vi "frontp_launch_default_subpanels.vi"(8 "error in (no error)":errorcluster, 11 "front_panel in":refnum<class "front_panel.lvclass">) -> (0 "error out":errorcluster, 3 "front_panel out":refnum<class "front_panel.lvclass">)   [LabVIEW 2015, in "front_panel.lvclass"]
uses:
  front_panel.lvclass
  Hardware Class/hardware_panel/Hardware_panel.lvclass
  hardware_caller_queue_numbers.ctl
  Detector_Class/detector_panel/Detector_panel.lvclass
  front_panel.lvclass/front_panel.ctl
  panel_class/panel.lvclass/panel.ctl
  panel_class/panel.lvclass
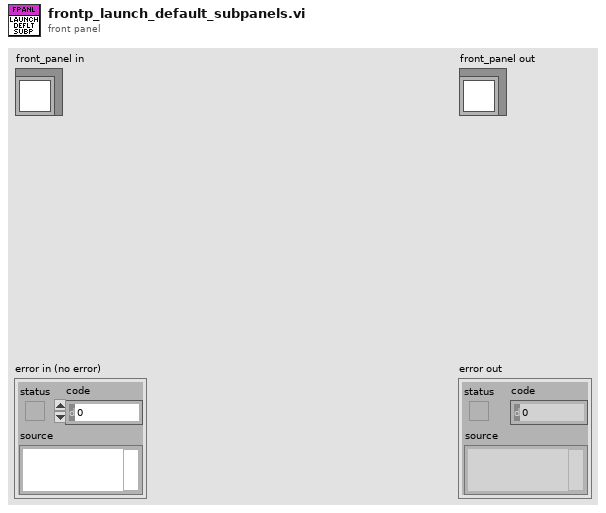
[diagram p1: front panel]
types:
  T1 = typedef "hardware_caller_queue_numbers.ctl" = enum16{"stage1", "stage2", "experiment", "detector"}
  T2 = typedef "gui_subpanel_references.ctl" = cluster{"Stage 1":refnum<vi>, "Stage 2":refnum<vi>, "Experiment":refnum<vi>, "Detector":refnum<vi>}
  T3 = typedef "hardware_seqs.ctl" = refnum<queue>[]
  T4 = typedef "ui_plot_references.ctl" = cluster{"plots":refnum<vi>, "chart":refnum<vi>, "graph":refnum<vi>, "map":refnum<vi>, "XY Graph":refnum<vi>}
  T5 = typedef "ui_user_events.ctl" = cluster{"update_xy_graph":refnum<user-event>, "update_graph":refnum<user-event>, "update_chart":refnum<user-event>, "update_map":refnum<user-event>, "event_loop_stop":refnum<user-event>, "keep_map":refnum<user-event>}
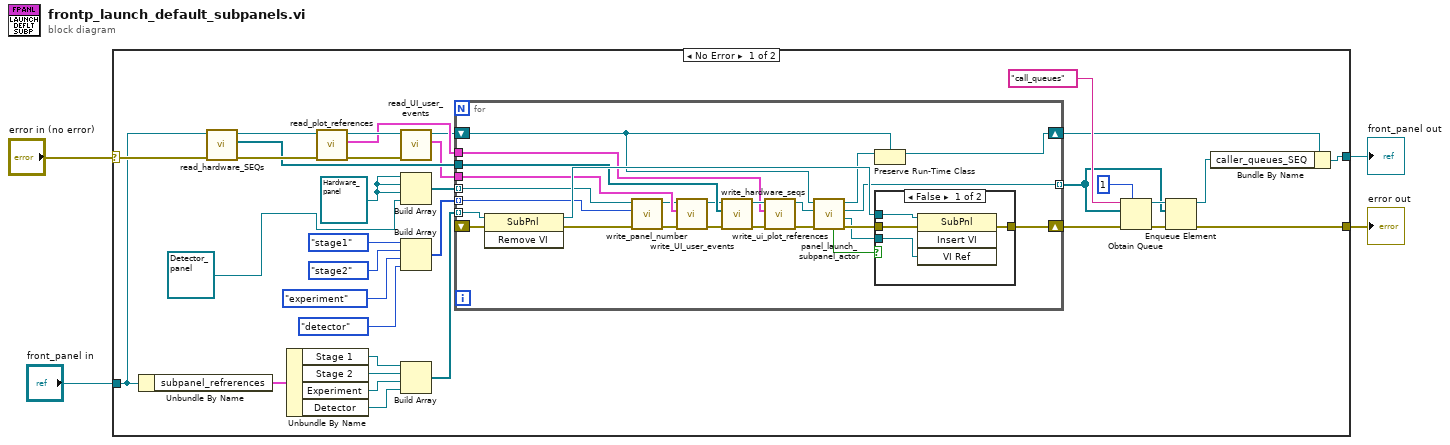
[diagram p0: block diagram]
diagram:
  n1 = case shown="No Error" "error in (no error)" {
    selector: "error in (no error)" -> [w15 w70]
    tunnel: [w26 w70] -> w3
    tunnel: [w28 w69] -> w1
    tunnel: "front_panel in" -> [w14 w69]
    frame No Error {
      w16 = refnum<class "Hardware_panel.lvclass"> refnum ("Hardware.lvclass")
      n2 = Unbundle By Name(w14) -> ("subpanel_refrerences"=w38:T2)
      n3 = call "read_hardware_SEQs.vi"("error in (no error)"=w15, "panel in"=w14) -> ("error out"=w13:errorcluster, "hardware_SEQs"=w9:T3, "panel out"=w12:refnum<class "front_panel.lvclass">)  [unwired: 7 in]
      n4 = Unbundle By Name(w38) -> ("Stage 1"=w37:refnum<vi>, "Stage 2"=w36:refnum<vi>, "Experiment"=w35:refnum<vi>, "Detector"=w34:refnum<vi>)
      n5 = call "read_plot_references.vi"("error in (no error)"=w13, "panel in"=w12) -> ("error out"=w10:errorcluster, "plot_references"=w8:T4, "panel out"=w11:refnum<class "front_panel.lvclass">)  [unwired: 7 in]
      n6 = call "read_UI_user_events.vi"("error in (no error)"=w10, "panel in"=w11) -> ("ui_user_events"=w7:T5, "panel out"=w6:refnum<class "front_panel.lvclass">)  [unwired: 7 in, 1 out]
      n7 = Build Array(w16, w16, w16, refnum<class "Detector_panel.lvclass"> refnum ("Detector_panel.lvclass")) -> (w17:refnum<class "panel.lvclass">[])
      n8 = Build Array(hardware_caller_queue_numbers."stage1" ("panel_number"), hardware_caller_queue_numbers."stage2" ("element"), hardware_caller_queue_numbers."experiment" ("element"), hardware_caller_queue_numbers."detector" ("element")) -> (w18:T1[])
      n9 = Build Array(w37, w36, w35, w34) -> (w33:refnum<vi>[])
      n10 = for {
        tunnel: w33 -> [w63] mode=indexing
        shift-right: [w60] -> w30
        shift-left: _ -> [w62]
        tunnel: w17 -> [w41] mode=indexing
        shift-right: [w53] -> w29
        shift-left: w6 -> [w54]
        tunnel: [w58] -> w24 mode=indexing
        tunnel: w9 -> [w47]
        tunnel: w18 -> [w39] mode=indexing
        tunnel: w8 -> [w48]
        tunnel: w7 -> [w44]
        n11 = invoke class="SubPnl" method="Remove VI"(reference=w63, error in=w62) -> (reference out=w61:refnum<vi>, error out=w43:errorcluster)  [unwired: 1 in, 1 out]
        n12 = call "write_panel_number.vi"("error in (no error)"=w43, "panel_number"=w39, "panel in"=w41) -> ("error out"=w42:errorcluster, "panel out"=w40:refnum<class "panel.lvclass">)  [unwired: 7 in]
        n13 = call "write_UI_user_events.vi"("error in (no error)"=w42, "ui_events"=w44, "panel in"=w40) -> ("error out"=w46:errorcluster, "panel out"=w45:refnum<class "panel.lvclass">)  [unwired: 7 in]
        n14 = call "write_hardware_seqs.vi"("error in (no error)"=w46, "hardware_SEQs"=w47, "panel in"=w45) -> ("error out"=w52:errorcluster, "panel out"=w50:refnum<class "panel.lvclass">)  [unwired: 7 in]
        n15 = call "write_ui_plot_references.vi"("error in (no error)"=w52, "plot_references"=w48, "panel in"=w50) -> ("error out"=w51:errorcluster, "panel out"=w49:refnum<class "panel.lvclass">)  [unwired: 7 in]
        n16 = call-dynamic "panel_launch_subpanel_actor.vi"("error in (no error)"=w51, "nested_panel"=w49, "caller_panel"=w54) -> ("error out"=w59:errorcluster, "subpanel_reference"=w57:refnum<vi>, "Nested Actor's Enqueuer"=w58:refnum<class "Message Enqueuer.lvclass">, "Caller Actor out"=w55:refnum<class "panel.lvclass">, "timed out?"=w56:bool)  [unwired: 4 in]
        n17 = Preserve Run-Time Class(object in=w55, 2:w54) -> (object out=w53:refnum<class "front_panel.lvclass">)  [unwired: 1 in, 1 out]
        n18 = case shown="False" w56 {
          tunnel: w61 -> [w67 _]
          tunnel: w59 -> [w66 w68]
          tunnel: [w65 w68] -> w60
          tunnel: w57 -> [w64 _]
          frame False {
            n19 = invoke class="SubPnl" method="Insert VI"(reference=w67, error in=w66, "VI Ref"=w64) -> (error out=w65:errorcluster)  [unwired: 1 in, 3 out]
          }
          frame True {
          }
        }
      }
      n20 = Obtain Queue(max queue size (-1, unlimited)=1, name (unnamed)="call_queues", element data type=w24, error in (no error)=w30) -> (queue out=w25:refnum<queue>, error out=w27:errorcluster)  [unwired: 1 in, 1 out]
      n21 = Enqueue Element(queue=w25, element=w24, error in (no error)=w27) -> (queue out=w23:refnum<queue>, error out=w26:errorcluster)  [unwired: 1 in, 1 out]
      n22 = Bundle By Name(cluster=w29, "caller_queues_SEQ"=w23) -> (w28:refnum<class "front_panel.lvclass">)
    }
    frame Error {
    }
  }
  "error out" <- w3
  "front_panel out" <- w1
